vi "加载病人.vi"(0 "connection information 2":path, 2 "输入身份证":string) -> (13 "语音测评":string, 14 "姓名":string[](array[string]), 15 "问卷调查":string, 16 "快速测查数据":string[](array[string]), 17 "左右耳结论":string[](array[string]), 18 "性别":string[](array[string]), 19 "身份证":string[](array[string]))   [LabVIEW 2013]
uses:
  <vilib>/addons/database/Connection.llb/DB Tools Open Connec (Path).vi
  <vilib>/addons/database/NI_Database_API.lvlib
panel:
  out "data":variant[][](array[variant])
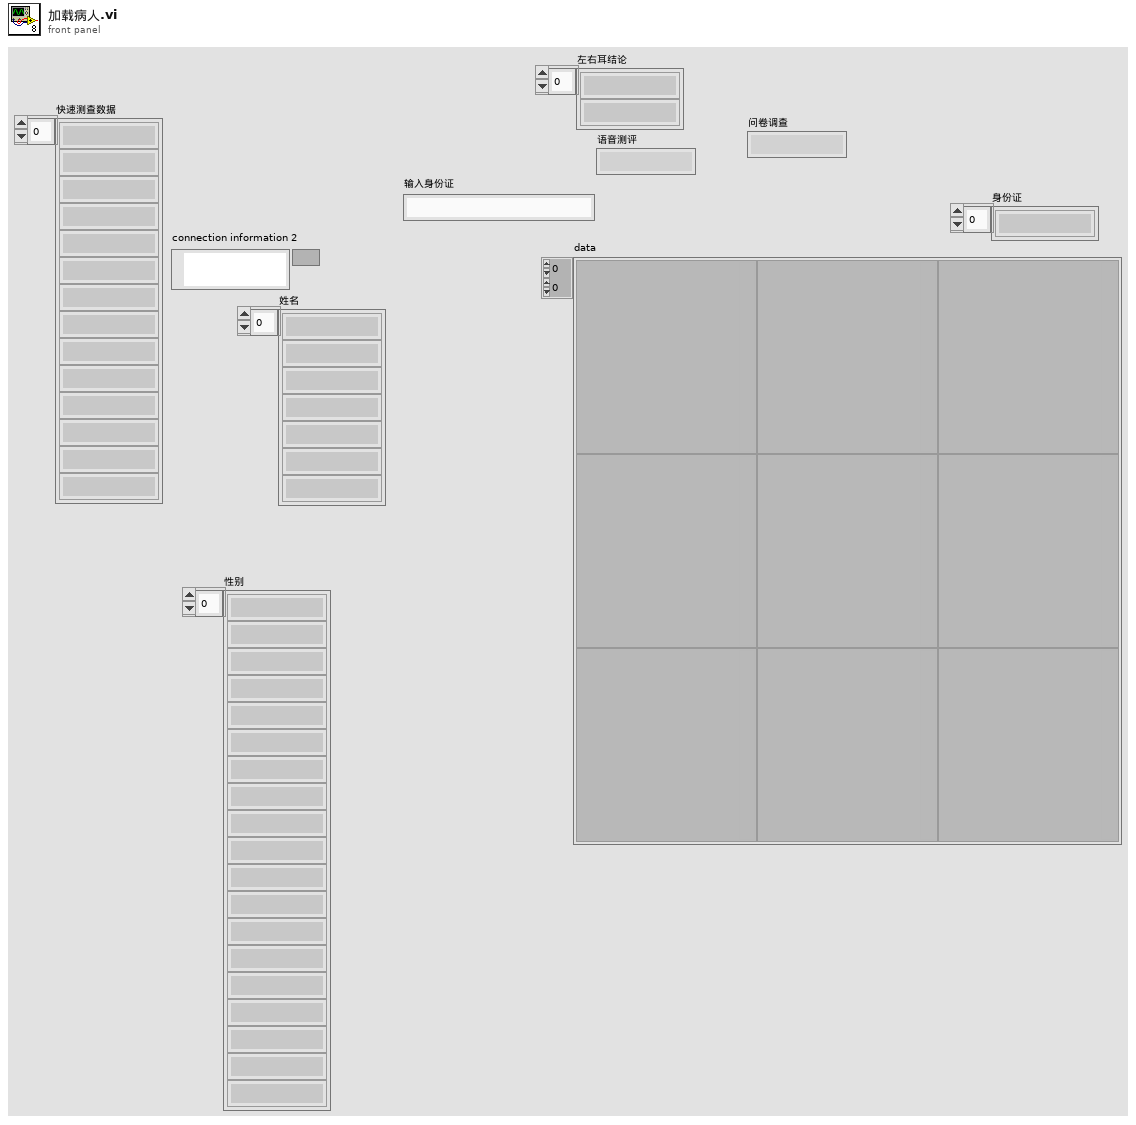
[diagram p1: front panel]
types:
  T1 = typedef "NI_Database_API.lvlib/Conn ObjectReference.ctl" = refnum<k1>
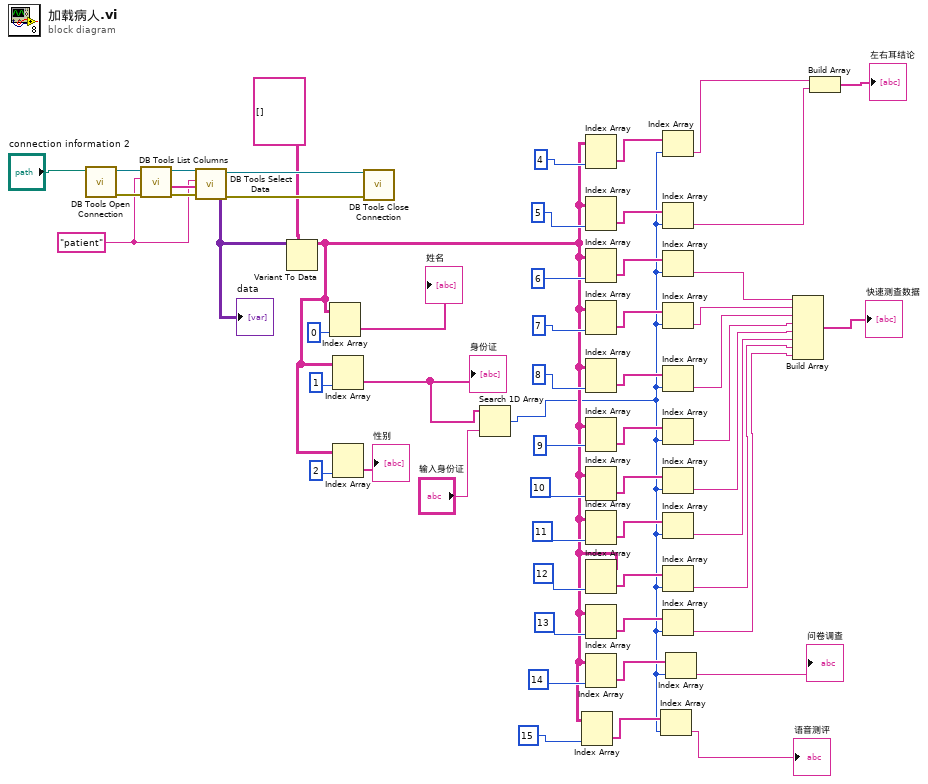
[diagram p0: block diagram]
diagram:
  w52 = "patient"
  n1 = call-poly <vilib>:"DB Tools Open Connection.vi"("connection information"="connection information 2") -> ("error out"=w53:errorcluster, "connection reference"=w57:T1)  [unwired: 7 in]
  n2 = call <vilib>:"DB Tools List Columns.vi"("error in (no error)"=w53, "table"=w52, "connection reference"=w57) -> ("error out"=w54:errorcluster, "columns"=w55:string[], "connection reference out"=w56:T1)  [unwired: 1 in, 1 out]
  n3 = call <vilib>:"DB Tools Select Data.vi"("error in (no error)"=w54, "columns"=w55, "table"=w52, "connection reference"=w56) -> ("error out"=w50:errorcluster, "data"=w49:variant[][], "connection reference out"=w51:T1)  [unwired: 2 in]
  "data" <- w49
  n4 = Variant To Data(type=string[][] [], Variant=w49) -> (data=w4:string[][])  [unwired: 1 in, 1 out]
  n5 = Index Array(array=w4, index (col)=0 ("禁用的索引 (列)")) -> (element=→"姓名":string[])  [unwired: 1 in]
  n6 = Index Array(array=w4, index (col)=1) -> (element=w42:string[])  [unwired: 1 in]
  "身份证" <- w42
  n7 = Index Array(array=w4, index (col)=2) -> (element=→"性别":string[])  [unwired: 1 in]
  n8 = call <vilib>:"DB Tools Close Connection.vi"("error in (no error)"=w50, "connection reference"=w51) -> ()  [unwired: 5 in, 1 out]
  n9 = Search 1D Array(1D array=w42, element="输入身份证") -> (index of element=w1:i32)  [unwired: 1 in]
  n10 = Index Array(array=w4, index (col)=15) -> (element=w3:string[])  [unwired: 1 in]
  n11 = Index Array(array=w4, index (col)=4) -> (element=w40:string[])  [unwired: 1 in]
  n12 = Index Array(array=w4, index (col)=5) -> (element=w28:string[])  [unwired: 1 in]
  n13 = Index Array(array=w4, index (col)=6) -> (element=w27:string[])  [unwired: 1 in]
  n14 = Index Array(array=w4, index (col)=7) -> (element=w26:string[])  [unwired: 1 in]
  n15 = Index Array(array=w4, index (col)=8) -> (element=w25:string[])  [unwired: 1 in]
  n16 = Index Array(array=w4, index (col)=9) -> (element=w24:string[])  [unwired: 1 in]
  n17 = Index Array(array=w4, index (col)=10) -> (element=w23:string[])  [unwired: 1 in]
  n18 = Index Array(array=w4, index (col)=11) -> (element=w22:string[])  [unwired: 1 in]
  n19 = Index Array(array=w4, index (col)=12) -> (element=w21:string[])  [unwired: 1 in]
  n20 = Index Array(array=w4, index (col)=13) -> (element=w20:string[])  [unwired: 1 in]
  n21 = Index Array(array=w4, index (col)=14) -> (element=w19:string[])  [unwired: 1 in]
  n22 = Index Array(array=w3, index=w1) -> (element=→"语音测评":string)
  n23 = Index Array(array=w40, index=w1) -> (element=w8:string)
  n24 = Index Array(array=w28, index=w1) -> (element=w7:string)
  n25 = Index Array(array=w27, index=w1) -> (element=w17:string)
  n26 = Index Array(array=w26, index=w1) -> (element=w16:string)
  n27 = Index Array(array=w25, index=w1) -> (element=w15:string)
  n28 = Index Array(array=w24, index=w1) -> (element=w14:string)
  n29 = Index Array(array=w23, index=w1) -> (element=w13:string)
  n30 = Index Array(array=w22, index=w1) -> (element=w12:string)
  n31 = Index Array(array=w21, index=w1) -> (element=w11:string)
  n32 = Index Array(array=w20, index=w1) -> (element=w10:string)
  n33 = Index Array(array=w19, index=w1) -> (element=→"问卷调查":string)
  n34 = Build Array(w17, w16, w15, w14, w13, w12, w11, w10) -> (→"快速测查数据":string[])
  n35 = Build Array(w8, w7) -> (→"左右耳结论":string[])
